vi "build.procElement.parse.vi"(11 "procElement in":variant) -> (0 "error out":errorcluster, 3 "UiBuildProcHead":T1)   [LabVIEW 2024]
uses:
  controls/UiProcHeader.ctl
  controls/typeProcVarientName.ctl
  Polymorphics/variantCtrlString.vi
  Polymorphics/variantCtrlBoolean.vi
  proc.util.validateParamExist.vi
  <vilib>/Utility/error.llb/Clear Errors.vi
  util.error.create.vi
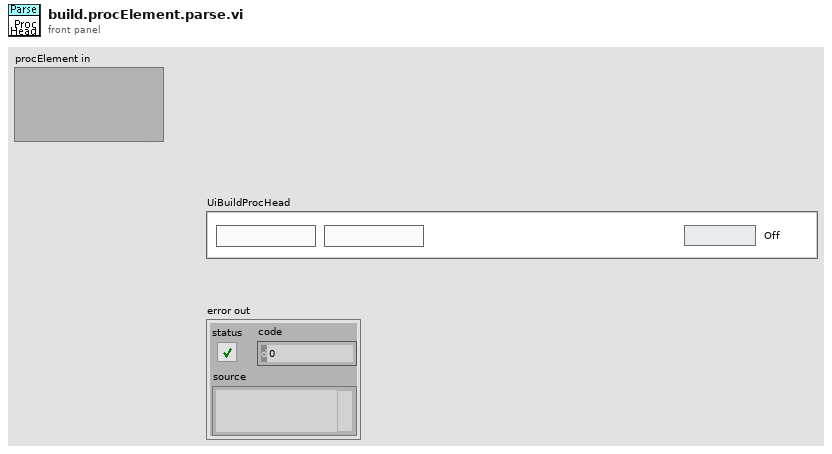
[diagram p1: front panel]
types:
  T1 = typedef "UiProcHeader.ctl" = cluster{"Procedure Name":string, "Running":bool, "tags":string}
  T2 = typedef "typeProcVarientName.ctl" = enum16{"procNameID", "procModuleID", "procPath", "procIsRunning", "procIndex", "procModule", "procRegisterNumeric", "procRegisterString", "procReport", "procReportPrev", "procCLK", "procStepPointer", "procType"}
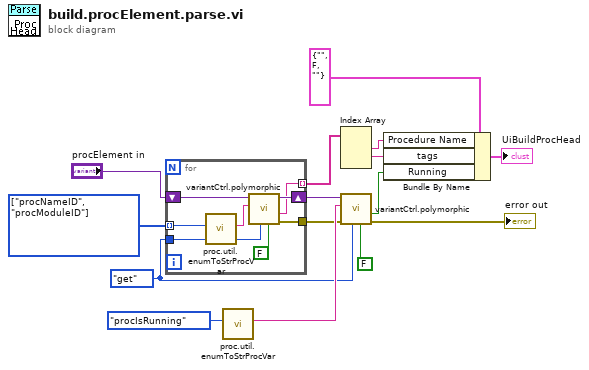
[diagram p0: block diagram]
diagram:
  w2 = enum16{"get", "set"}."get" ("menu in (get)")
  w7 = T2[] [enum."procNameID", enum."procModuleID"] items=["procNameID", "procModuleID", "procPath", "procIsRunning", "procIndex", "procModule", "procRegisterNumeric", "procRegisterString", "procReport", "procReportPrev", "procCLK", "procStepPointer", "procType"] ("Proc var")
  n1 = for {
    tunnel: w7 -> [w22] mode=indexing
    tunnel: [w19] -> w3
    tunnel: w2 -> [w18]
    shift-right: [w20] -> w6
    shift-left: "procElement in" -> [w23]
    tunnel: [w17] -> w11 mode=indexing
    n2 = call "proc.util.enumToStrProcVar.vi"("Proc var"=w22) -> ("String"=w21:string)  [unwired: 10 in]
    n3 = call-poly "variantCtrl.polymorphic.vi"("isRequired (T)"=FALSE, "menu in (get)"=w18, "name in"=w21, "Step in"=w23) -> ("error out"=w19:errorcluster, "String Value"=w17:string, "Step out"=w20:variant)  [unwired: 4 in, 1 out]
  }
  n4 = call "proc.util.enumToStrProcVar.vi"("Proc var"=typeProcVarientName."procIsRunning") -> ("String"=w4:string)  [unwired: 10 in]
  n5 = Index Array(array=w11) -> (element #1=w12:string, element #2=w13:string)  [unwired: 3 in, 1 out]
  n6 = call-poly "variantCtrl.polymorphic.vi"("isRequired (T)"=FALSE, "menu in (get)"=w2, "error in"=w3, "name in"=w4, "variant in"=w6) -> ("error out"=→"error out":errorcluster, "Boolean Value out"=w14:bool)  [unwired: 3 in, 2 out]
  n7 = Bundle By Name(cluster=T1 {"Procedure Name"="", "Running"=FALSE, "tags"=""} ("UiBuildProcHead 3"), "Procedure Name"=w12, "tags"=w13, "Running"=w14) -> (→"UiBuildProcHead":T1)
